vi "二维数组与表格字符串相互转换.vi"() -> ()   [LabVIEW 2010]
panel:
  out "数组":string[][](array[string])
  out "字符串":string
  in  "输组":string[][](array[string])
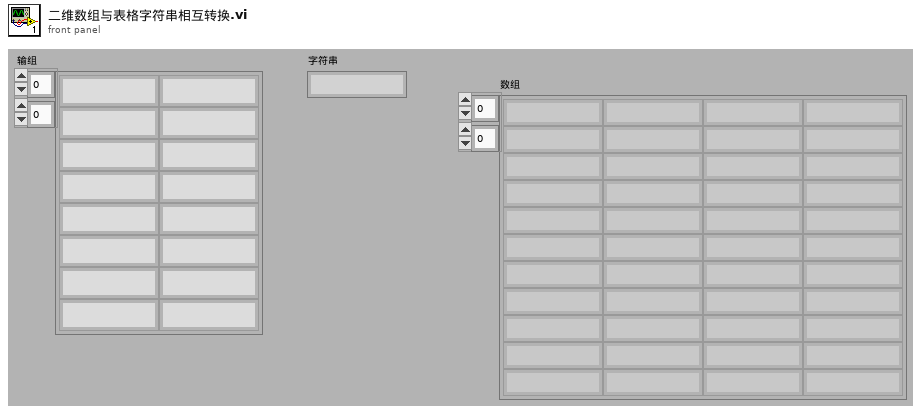
[diagram p1: front panel]
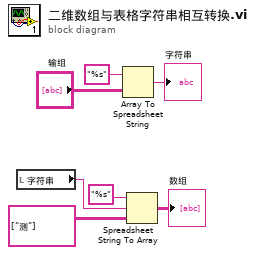
[diagram p0: block diagram]
diagram:
  n1 = local read "字符串"() -> (w4:string)
  n2 = Array To Spreadsheet String(array="输组", 3:"%s" ("格式字符串")) -> (spreadsheet string=→"字符串":string)  [unwired: 1 in]
  n3 = Spreadsheet String To Array(format string="%s" ("格式字符串"), spreadsheet string=w4, array type (2D Dbl)=string[][] [["测"]] ("数组类型(2D String)")) -> (array=→"数组":string[][])  [unwired: 1 in]
